vi "mtoe.vi"(11 "m":dbl) -> (3 "e":dbl)   [LabVIEW 2019]
panel:
  # "e"
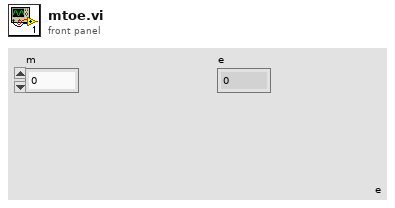
[diagram p1: front panel]
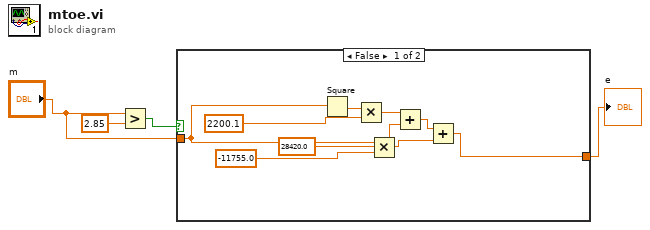
[diagram p0: block diagram]
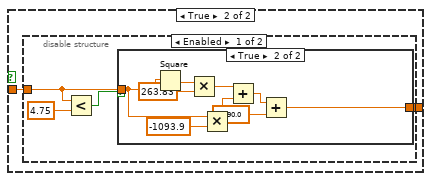
[diagram p2: hidden frame]
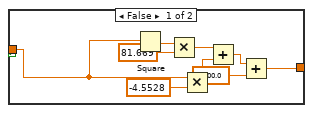
[diagram p3: hidden frame]
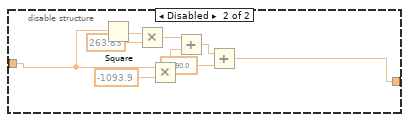
[diagram p4: hidden frame]
diagram:
  n1 = Greater?(x="m", y=2.85) -> (0:w3:bool)
  n2 = case shown="False" w3 {
    tunnel: "m" -> [w6 w14]
    tunnel: [w5 w15] -> w1
    frame False {
      n3 = Square(x=w6) -> (x^2=w12:dbl)
      n4 = Multiply(x=w12, y=2200.1) -> (x*y=w13:dbl)
      n5 = Multiply(x=w6, y=-11755.0) -> (x*y=w10:dbl)
      n6 = Add(x=w13, y=w10) -> (x+y=w8:dbl)
      n7 = Add(x=w8, y=28420.0) -> (x+y=w5:dbl)
    }
    frame True {
      n8 = disable-structure shown="Enabled" {
        disable-tunnel: [w19 w38] -> w15
        disable-tunnel: w14 -> [w17 w39]
        frame Enabled {
          n9 = Less?(x=w17, y=4.75) -> (x < y?=w16:bool)
          n10 = case shown="True" w16 {
            tunnel: [w21 w30] -> w19
            tunnel: w17 -> [w20 w29]
            frame False {
              n11 = Square(x=w20) -> (x^2=w27:dbl)
              n12 = Multiply(x=w27, y=81.669) -> (x*y=w28:dbl)
              n13 = Multiply(x=w20, y=-4.5528) -> (x*y=w25:dbl)
              n14 = Add(x=w28, y=w25) -> (x+y=w23:dbl)
              n15 = Add(x=w23, y=11800.0) -> (x+y=w21:dbl)
            }
            frame True {
              n16 = Square(x=w29) -> (x^2=w36:dbl)
              n17 = Multiply(x=w36, y=263.83) -> (x*y=w37:dbl)
              n18 = Multiply(x=w29, y=-1093.9) -> (x*y=w34:dbl)
              n19 = Add(x=w37, y=w34) -> (x+y=w32:dbl)
              n20 = Add(x=w32, y=13690.0) -> (x+y=w30:dbl)
            }
          }
        }
        frame Disabled {
          n21 = Square(x=w39) -> (x^2=w45:dbl)
          n22 = Multiply(x=w45, y=263.83) -> (x*y=w46:dbl)
          n23 = Multiply(x=w39, y=-1093.9) -> (x*y=w43:dbl)
          n24 = Add(x=w46, y=w43) -> (x+y=w41:dbl)
          n25 = Add(x=w41, y=13690.0) -> (x+y=w38:dbl)
        }
      }
    }
  }
  "e" <- w1
